vi "STD浊度_获取温度和测量值.vi"(8 "error in (no error)":errorcluster caption="错误输入（无错误）", 11 "MB session in":refnum<class "MB_Master.lvclass">) -> (0 "error out":errorcluster caption="错误输出", 2 "STD浊度":cluster{"温度测量值":sgl, "浊度测量值":sgl, "信号值":sgl}, 3 "MB session out":refnum<class "MB_Master.lvclass">)   [LabVIEW 2016, in "斯坦道多参数.lvlib"]
uses:
  <vilib>/Plasmionique/MB Master/MB_Master/MB_Master.lvclass
  <vilib>/Plasmionique/MB Master/MB Master.lvlib
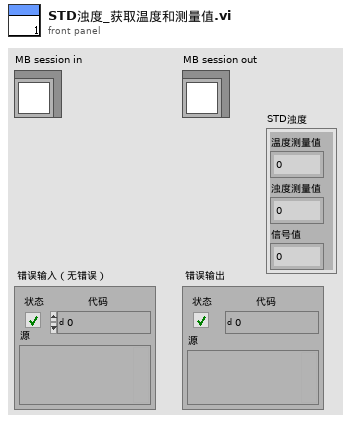
[diagram p1: front panel]
types:
  T1 = cluster{"pH":u32, "DO":u32, "Cond":u32, "Turb":u32, "叶绿素a":u32, "藻密度":u32, "ORP":u32, "COD":u32, "氯化物":u32, "氨氮":u32, "水中油":u32, "悬浮物":u32, "余氯":u32}
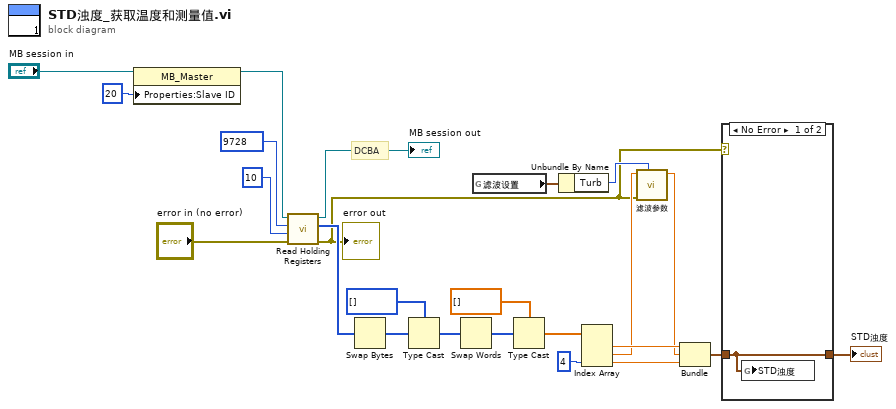
[diagram p0: block diagram]
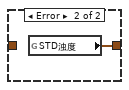
[diagram p2: hidden frame]
diagram:
  # "DCBA"
  n1 = property class="MB_Master"(reference="MB session in", "Properties:Slave ID"=u16 20 ("y")) -> (reference out=w16:refnum<class "MB_Master.lvclass">)  [unwired: 1 in, 1 out]
  n2 = call <vilib>:"Read Holding Registers.vi"("error in (no error)"="error in (no error)", "quantity"=u16 10, "starting address"=u16 9728, "MB session in"=w16) -> ("error out"=w4:errorcluster, "Registers"=w14:u16[], "MB session out"=→"MB session out":refnum<class "MB_Master.lvclass">)  [unwired: 5 in]
  "error out" <- w4
  n3 = Swap Bytes(anything=w14) -> (byte swapped=w13:u16[])
  n4 = Type Cast(type=u32[] [] ("数组 2"), x=w13) -> (*(type *) &x=w20:u32[])
  n5 = Swap Words(1:w20) -> (0:w22:u32[])
  n6 = global read "断电保存变量.vi" "滤波设置"() -> (w6:T1)
  n7 = Type Cast(type=sgl[] [] ("数组 2"), x=w22) -> (*(type *) &x=w18:sgl[])
  n8 = Unbundle By Name(w6) -> ("Turb"=w5:u32)
  n9 = Index Array(array=w18, index #3=4 ("索引")) -> (element #1=w12:sgl, element #2=w8:sgl, element #3=w2:sgl)  [unwired: 2 in]
  n10 = call "滤波参数.vi"("滤波次数"=w5, "error in (no error)"=w4, "x"=w8) -> ("mode"=w7:dbl)  [unwired: 7 in, 1 out]
  n11 = Bundle("数值"=w12, "mode"=w7, "数值"=w2) -> (w11:cluster{"数值":sgl, "mode":dbl, "数值":sgl})  [unwired: 1 in]
  n12 = case shown="No Error" w4 {
    tunnel: w11 -> [w25 _]
    tunnel: [w25 w26] -> w1
    frame No Error {
      n13 = global write "禹山过程全局变量.vi" "STD浊度"(w25) -> ()
    }
    frame Error {
      n14 = global read "禹山过程全局变量.vi" "STD浊度"() -> (w26:cluster{"温度测量值":sgl, "浊度测量值":sgl, "信号值":sgl})
    }
  }
  "STD浊度" <- w1
